vi "fronts32.vi"(3 "IN":u32 format="%x") -> (0 "FALL":u32 format="%x", 1 "RAISE":u32 format="%x")   [LabVIEW 2019, in "Logik.lvlib"]
uses:
  Logik.lvlib
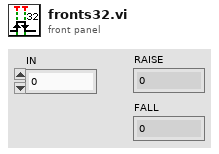
[diagram p1: front panel]
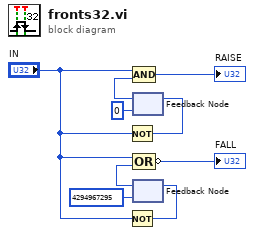
[diagram p0: block diagram]
diagram:
  n1 = Not(x="IN") -> (.not. x?=w9:u32)
  n2 = Not(x="IN") -> (.not. x?=w7:u32)
  n3 = feedback #1(u32 0) -> (w8:u32)
  n4 = Compound Arithmetic op=AND("IN", w8) -> (→"RAISE":u32)
  n5 = feedback-in #1(w9) -> ()
  n6 = feedback #2(u32 4294967295) -> (w6:u32)
  n7 = Compound Arithmetic op=OR("IN", w6) -> (invert →"FALL":u32)
  n8 = feedback-in #2(w7) -> ()
